vi "Convert to padded ROI index string.vi"(11 "ROI number":i32=3) -> (2 "ROI index string padded with zeroes":string)   [LabVIEW 2013]
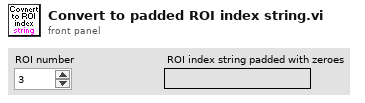
[diagram p1: front panel]
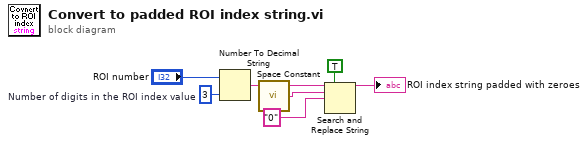
[diagram p0: block diagram]
diagram:
  w7 = i16 3  # Number of digits in the ROI index value
  n1 = Number To Decimal String(number="ROI number", width (-)=w7) -> (decimal integer string=w5:string)
  n2 = call <vilib>:"Space Constant.vi"() -> ("String"=w2:string)
  n3 = Search and Replace String(replace all?=TRUE ("replace all? (F)"), input string=w5, search string=w2, replace string="0") -> (result string=→"ROI index string padded with zeroes":string)  [unwired: 4 in, 3 out]
